vi "Read motion magic constants from config.vi"(8 "error in":errorcluster, 11 "Settings":variant) -> (0 "error out":errorcluster, 2 "Motion Magic Constants":T1, 3 "Settings out":variant)   [LabVIEW 2019, in "DriveOld.lvlib" / "Drive.lvclass"]
doc: "This VI reads the motion magic constants from the configuration variant."
uses:
  Drive.lvclass
  Controls/Motion Magic Constants.ctl
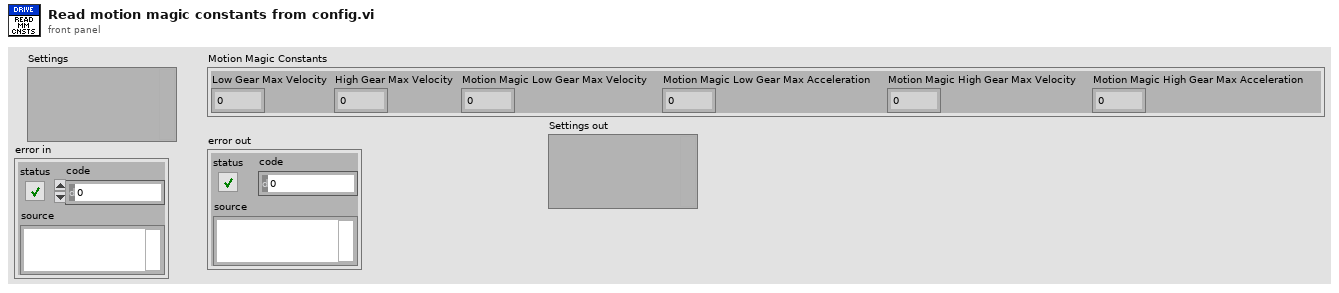
[diagram p1: front panel]
types:
  T1 = typedef "DriveOld.lvlib/Drive.lvclass/Motion Magic Constants.ctl" = cluster{"Low Gear Max Velocity":u32, "High Gear Max Velocity":u32, "Motion Magic Low Gear Max Velocity":u32, "Motion Magic Low Gear Max Acceleration":u32, "Motion Magic High Gear Max Velocity":u32, "Motion Magic High Gear Max Acceleration":u32}
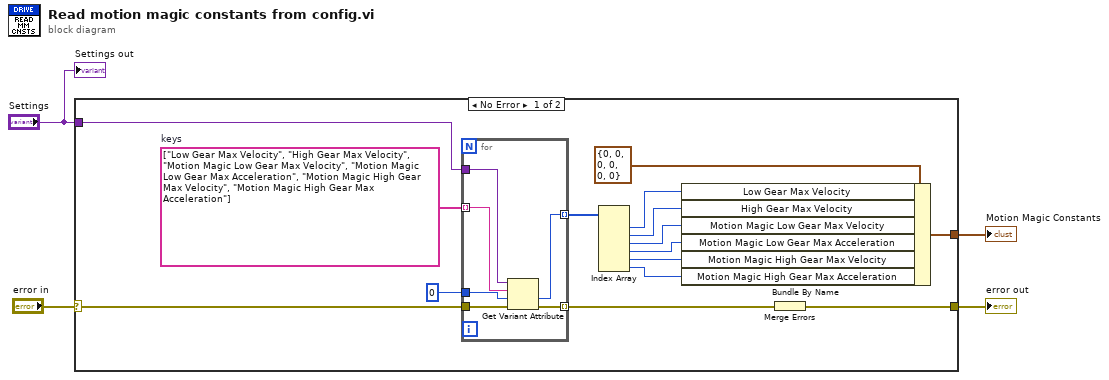
[diagram p0: block diagram]
diagram:
  n1 = case shown="No Error" "error in" {
    selector: "error in" -> [w5 w26]
    tunnel: [w19 w26] -> w4
    tunnel: "Settings" -> [w18 _]
    tunnel: [w7 _] -> w2
    frame No Error {
      w17 = string[] ["Low Gear Max Velocity", "High Gear Max Velocity", "Motion Magic Low Gear Max Velocity", "Motion Magic Low Gear Max Acceleration", "Motion Magic High Gear Max Velocity", "Motion Magic High Gear Max Acceleration"]  # keys
      n2 = for {
        tunnel: w18 -> [w25]
        tunnel: [w24] -> w8 mode=indexing
        tunnel: u32 0 ("Low Gear Max Velocity") -> [w23]
        tunnel: [w22] -> w16 mode=indexing
        tunnel: w17 -> [w21] mode=indexing
        tunnel: w5 -> [w20]
        n3 = Get Variant Attribute(Variant=w25, name=w21, default value (empty Variant)=w23, error in=w20) -> (value=w24:u32, error out=w22:errorcluster)  [unwired: 2 out]
      }
      n4 = Index Array(array=w8) -> (element #1=w10:u32, element #2=w11:u32, element #3=w12:u32, element #4=w13:u32, element #5=w14:u32, element #6=w15:u32)  [unwired: 6 in]
      n5 = Bundle By Name(cluster=T1 {"Low Gear Max Velocity"=0, "High Gear Max Velocity"=0, "Motion Magic Low Gear Max Velocity"=0, "Motion Magic Low Gear Max Acceleration"=0, "Motion Magic High Gear Max Velocity"=0, "Motion Magic High Gear Max Acceleration"=0} ("Motion Magic Constants"), "Low Gear Max Velocity"=w10, "High Gear Max Velocity"=w11, "Motion Magic Low Gear Max Velocity"=w12, "Motion Magic Low Gear Max Acceleration"=w13, "Motion Magic High Gear Max Velocity"=w14, "Motion Magic High Gear Max Acceleration"=w15) -> (w7:T1)
      n6 = Merge Errors(w16) -> (w19:errorcluster)
    }
    frame Error {
    }
  }
  "error out" <- w4
  "Motion Magic Constants" <- w2
  "Settings out" <- "Settings"
